vi "UIEnableyesnoo.vi"(0 "CmdLib In":refnum<k24>, 5 "Status:":refnum<vi>, 7 "UI":T1, 9 "Device Array":T2(array[cluster]), 11 "error in":errorcluster) -> (15 "error out":errorcluster)   [LabVIEW 2021]
uses:
  C:/Program Files/New Focus/New Focus Picomotor Application/Samples/LabVIEW/Model 8742/LabVIEW 2009/CmdLib.dll
  Program Files/New Focus/New Focus Picomotor Application/Samples/LabVIEW/Model 8742/LabVIEW 2009/CmdLib.dll
  Global Variablesyes.vi
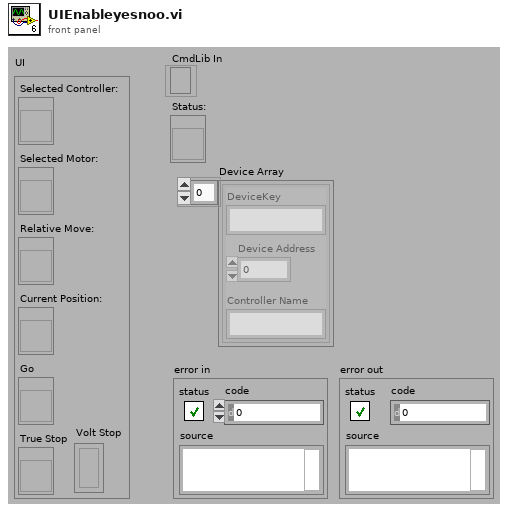
[diagram p1: front panel]
types:
  T1 = cluster{"Selected Controller:":refnum<vi>, "Selected Motor:":refnum<vi>, "Relative Move:":refnum<vi>, "Current Position:":refnum<vi>, "Go":refnum<vi>, "True Stop":refnum<vi>, "Volt Stop":refnum<vi>}
  T2 = cluster{"DeviceKey":string, "Device Address":i32, "Controller Name":string}[]
  T3 = enum8{"Enabled", "Disabled", "Disabled and Grayed Out"}
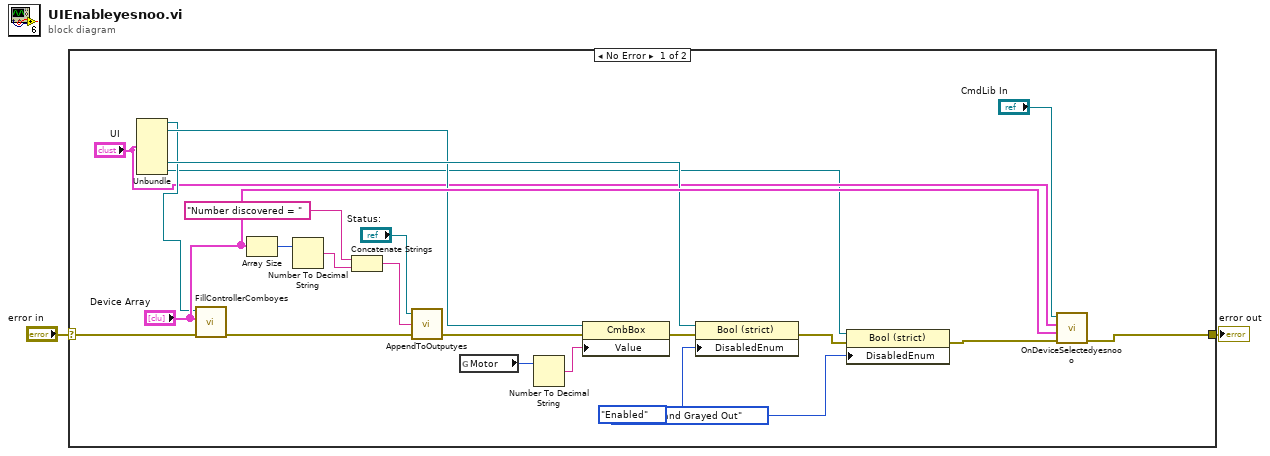
[diagram p0: block diagram]
diagram:
  n1 = case shown="No Error" "error in" {
    selector: "error in" -> [w19 w26]
    tunnel: [w21 w26] -> w2
    frame No Error {
      n2 = Unbundle("UI") -> ("Selected Controller:"=w8:refnum<vi>, "Selected Motor:"=w9:refnum<vi>, "True Stop"=w10:refnum<vi>, "Volt Stop"=w4:refnum<vi>)  [unwired: 3 out]
      n3 = call "FillControllerComboyes.vi"("error in (no error)"=w19, "Device Array"="Device Array", "Selected Controller:"=w8) -> ("error out"=w18:errorcluster)  [unwired: 8 in]
      n4 = Array Size(array="Device Array") -> (size(s)=w20:i32)
      n5 = Number To Decimal String(number=w20) -> (decimal integer string=w23:string)  [unwired: 1 in]
      n6 = Concatenate Strings("Number discovered = " ("string"), w23) -> (w25:string)
      n7 = call "AppendToOutputyes.vi"("error in"=w18, "Input String"=w25, "Output Refnum In"="Status:") -> ("error out"=w13:errorcluster)  [unwired: 1 in, 1 out]
      n8 = global read "Global Variablesyes.vi" "Motor"() -> (w16:i32)
      n9 = Number To Decimal String(number=w16) -> (decimal integer string=w17:string)  [unwired: 1 in]
      n10 = property class="CmbBox"(reference=w9, error in=w13, "Value"=w17) -> (error out=w11:errorcluster)  [unwired: 1 out]
      n11 = property class="Bool (strict)"(reference=w10, error in=w11, "DisabledEnum"=T3."Enabled" ("Disabled")) -> (error out=w6:errorcluster)  [unwired: 1 out]
      n12 = property class="Bool (strict)"(reference=w4, error in=w6, "DisabledEnum"=T3."Disabled and Grayed Out" ("Disabled")) -> (error out=w5:errorcluster)  [unwired: 1 out]
      n13 = call "OnDeviceSelectedyesnooo.vi"("error in"=w5, "Device Array"="Device Array", "UI"="UI", "CmdLib In"="CmdLib In") -> ("error out"=w21:errorcluster)  [unwired: 7 in]
    }
    frame Error {
    }
  }
  "error out" <- w2
